vi "ARD-LTC2499_EEPROM.vi"   [LabVIEW 2014]
doc: "Demonstrates how to read and write data to 24AA025E48 2Kb Serial EEPROM ."
uses:
  QwaveSys_Interface/QwaveSys_Interface.lvlib
  PWS_ESP8266/PWS_ESP8266.lvlib
panel:
  # "Overview: Demonstrates how to read EEPROM data from I2C 24AA02E48 serial EEPROM EUI-48 chip. This example using ARD-LTD2499 shiled that has onboard \"24AA02E48\" chip, Refer at this link: http://www.iascaled.com/store/ARD-LTC2499\nRequirements: LabVIEW Full Development System,Arduino Compatible Compiler for LabVIEW,Programmable Wireless Stamp (PWS) Library.\nInstructions:\n1. Wire the ARD-LTC2499 power pins to VCC and GND and the I2C pins to the Pmod I2C interface.  Note that on an PWS board, the I2C pins are on GPIO2 (SDA) and GPIO14 (SCL) \n2. If this example has been loaded from the Arduino Compatible Compiler for LabVIEW, simply select Compile and Download.  Otherwise, open Tools>Arduino Compatible Compiler for LabVIEW in LabVIEW, then select File>Load VI, and select this VI and then Compile and Download.\n3. Open \"Serial Monitor\" by select \"Tools>Serial Monitor\" and select baud rate to 9600.\n4. Observe the data that written to EEPROM  being print out on serial port monitor.\n5. Observe the data that read from EEPROM  being print out on serial port monitor.\n6. Observe the data that read from EUI48  being print out on serial port monitor.\n\n#NOTE: \nThe 24AA02E48 is a 2k I2C serial EEPROM EUI-48 node identity by Microchip technologies. The EEPROM includes pre-programmed globally unique 48-bit node address for applications that require unique identification.\nrefer: http://ww1.microchip.com/downloads/en/DeviceDoc/22124D.pdf"
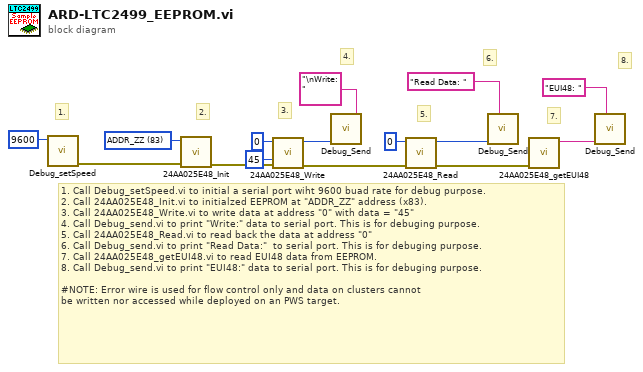
[diagram p0: block diagram]
diagram:
  w15 = u8 83 items=["ADDR_00"=80, "ADDR_0Z"=81, "ADDR_Z0"=82, "ADDR_ZZ"=83] ("Address")
  # "1. Call Debug_setSpeed.vi to initial a serial port wiht 9600 buad rate for debug purpose.\n2. Call 24AA025E48_Init.vi to initialzed EEPROM at \"ADDR_ZZ\" address (x83).\n3. Call 24AA025E48_Write.vi to write data at address \"0\" with data = \"45\"\n4. Call Debug_send.vi to print \"Write:\" data to serial port. This is for debuging purpose.\n5. Call 24AA025E48_Read.vi to read back the data at address \"0\"\n6. Call Debug_send.vi to print \"Read Data:\"  to serial port. This is for debuging purpose.\n7. Call 24AA025E48_getEUI48.vi to read EUI48 data from EEPROM.\n8. Call Debug_send.vi to print \"EUI48:\" data to serial port. This is for debuging purpose.\n\n#NOTE: Error wire is used for flow control only and data on clusters cannot\nbe written nor accessed while deployed on an PWS target."
  # "8."
  # "7."
  # "6."
  # "5."
  # "4."
  # "3."
  # "2."
  # "1."
  n1 = call "Debug_setSpeed.vi"("Speed"=u32 9600) -> ("error out"=w10:errorcluster)  [unwired: 10 in]
  n2 = call "24AA025E48_Init.vi"("error in (no error)"=w10, "Address"=w15) -> ("error out"=w14:errorcluster)  [unwired: 9 in]
  n3 = call "24AA025E48_Write.vi"("error in (no error)"=w14, "Data"=u8 45, "Address"=u16 0) -> ("error out"=w13:errorcluster, "error"=w7:u8)  [unwired: 7 in]
  n4 = call "Debug_Send.vi"("Name"="\nWrite: ", "DATA"=w7) -> ()  [unwired: 10 in]
  n5 = call "24AA025E48_Read.vi"("error in (no error)"=w13, "Address"=u16 0) -> ("error out"=w3:errorcluster, "Data"=w4:u8)  [unwired: 8 in]
  n6 = call "Debug_Send.vi"("Name"="Read Data: ", "DATA"=w4) -> ()  [unwired: 10 in]
  n7 = call "24AA025E48_getEUI48.vi"("error in (no error)"=w3) -> ("EUI48"=w2:string)  [unwired: 9 in, 1 out]
  n8 = call "Debug_Send.vi"("Name"="EUI48: ", "DATA"=w2) -> ()  [unwired: 10 in]
